vi "Find Collapsed Nodes.vi"(11 "TreeControl in":refnum<vi>) -> (0 "error out":errorcluster, 2 "tags of collapsed nodes":string[](array[string]))   [LabVIEW 2013]
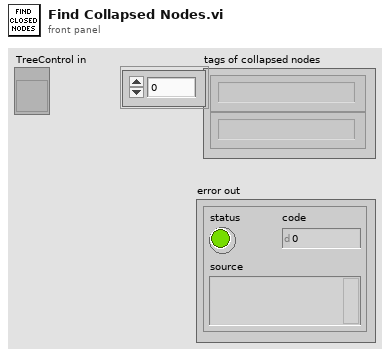
[diagram p1: front panel]
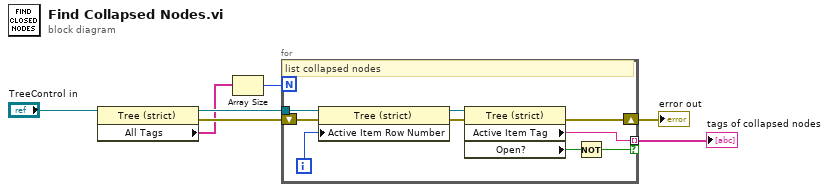
[diagram p0: block diagram]
diagram:
  n1 = property class="Tree (strict)"(reference="TreeControl in") -> (reference out=w6:refnum<vi>, error out=w3:errorcluster, "All Tags"=w2:string[])  [unwired: 1 in]
  n2 = Array Size(array=w2) -> (size(s)=w1:i32)
  n3 = for {
    N: w1 -> [_]
    tunnel: w6 -> [w15]
    tunnel: [w10] -> w5 mode=indexing if=w9
    shift-right: [w11] -> w4
    shift-left: w3 -> [w13]
    i -> [w8]
    # "list collapsed nodes"
    n4 = property class="Tree (strict)"(reference=w15, error in=w13, "Active Item Row Number"=w8) -> (reference out=w16:refnum<vi>, error out=w12:errorcluster)
    n5 = property class="Tree (strict)"(reference=w16, error in=w12) -> (error out=w11:errorcluster, "Active Item Tag"=w10:string, "Open?"=w14:bool)  [unwired: 1 out]
    n6 = Not(x=w14) -> (.not. x?=w9:bool)
  }
  "tags of collapsed nodes" <- w5
  "error out" <- w4
